vi "LVFunction_Imop_HAS file_GetSoftwareInformation.vi"(0 "HAS file path":path, 11 "error in (no error)":errorcluster) -> (4 "HasoModel":string, 6 "HasoSerial Number":string, 8 "SoftwareOptionsList":string[](array[string]), 13 "comments":string, 14 "session_name":string, 15 "error out":errorcluster)   [LabVIEW 2018]
doc: "Get informations from HasoData object.\n\n<B>HasoDataIn</B> : HasoData object.\n<B>HasoDataOut</B> : HasoData object.\n<B>haso_model</B> : Sensor model.\n<B>haso_serial_number</B> : Haso serial number.\n<B>camera_serial_number</B> : Camera serial number.\n<B>revisions</B> : Revision number.\n<B>lower_calibration_wl</B> : Lower calibration wavelength (nm).\n<B>upper_calibration_wl</B> : Upper calibration wavelength (nm).\n<B>exposure_time_requested</B> : Exposure duration requested, in microsecond.\n<B>exposure_time_applied</B> : Exposure duration applied, in microsecond.\n<B>nb_summed_images</B> : Number of summed images.\n<B>time_stamp</B> : Timestamp.\n<B>is_background_removed</B> : Background removed value.\n<B>is_smearing_removed</B> : Smearing removed value.\n<B>wavelength_nm</B> : Source wavelength (nm).\n<B>session_name</B> : Session name.\n<B>trigger_type</B> : Trigger mode.\n<B>comments</B> : Comments.\n<B>max_level</B> : Max level value.\n<B>start_subpupil</B> : Start subpupil position (um)\n<B>denoising_strength</B> : Sensitivity of spot detection (between 0 and 1). Modulates noise management\n when computing slopes on summed images.\n * 0 : Release constraint on noise to detect as much sub-pupils as possible.\n * 1 : Do not take into account the noise reduction caused by summing.\n<B>ErrorIn </B> : Error\n<B>ErrorOut </B> : Error"
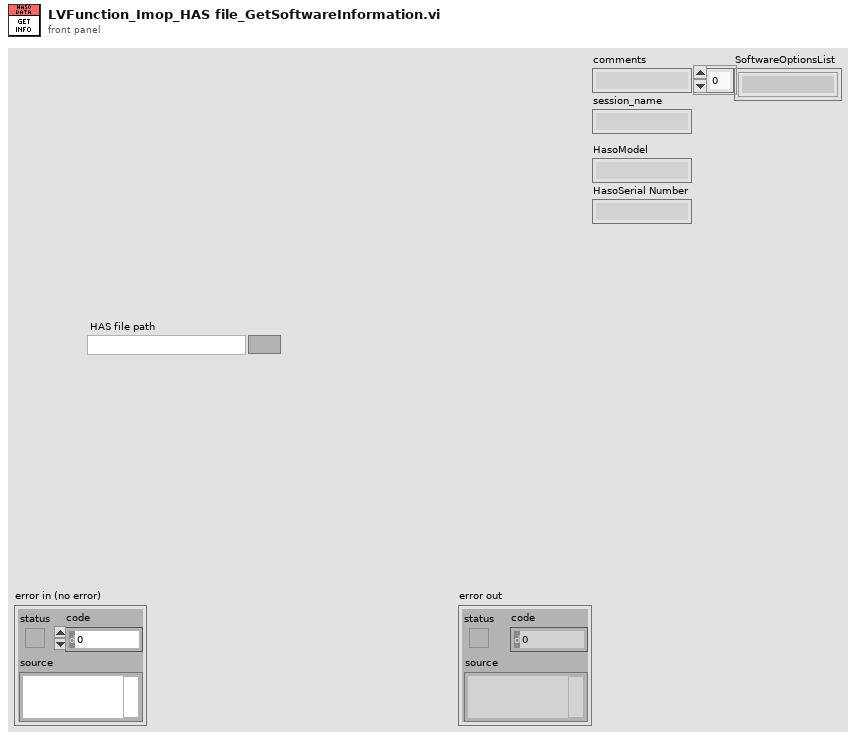
[diagram p1: front panel]
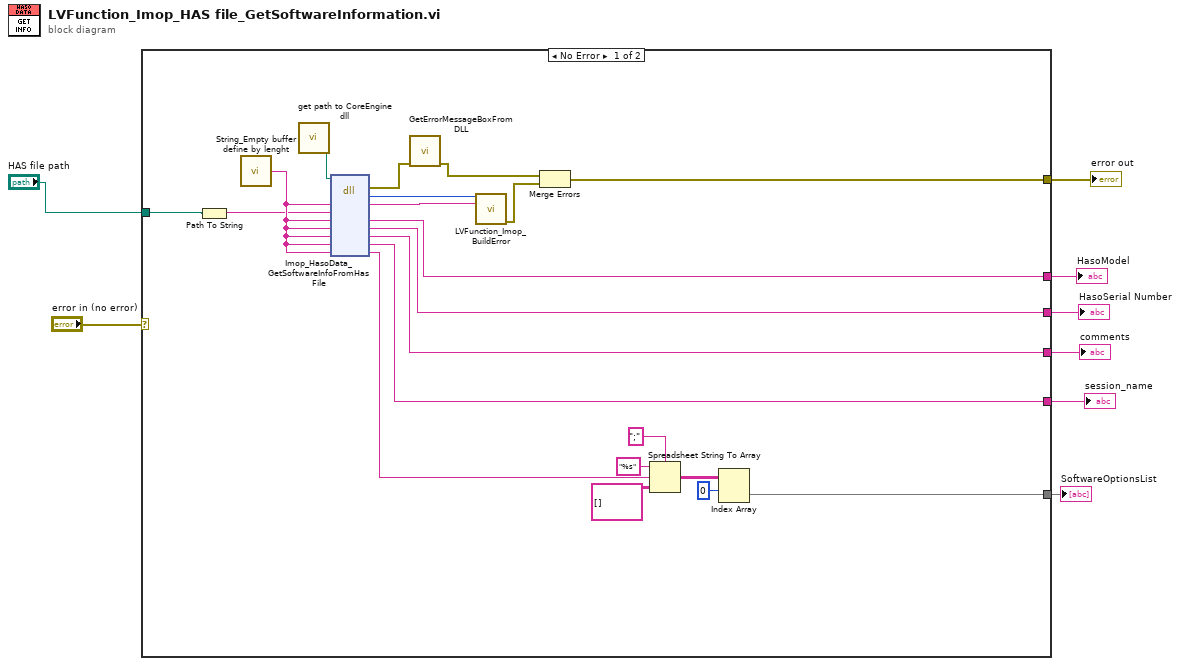
[diagram p0: block diagram]
diagram:
  n1 = case shown="No Error" "error in (no error)" {
    selector: "error in (no error)" -> [_ w30]
    tunnel: [w23 w30] -> w7
    tunnel: [w21 _] -> w6
    tunnel: [w20 _] -> w5
    tunnel: "HAS file path" -> [w19 _]
    tunnel: [w17 _] -> w3
    tunnel: [w16 _] -> w2
    tunnel: [w9 _] -> w1
    frame No Error {
      n2 = Path To String(path=w19) -> (string=w18:string)
      n3 = call "String_Empty buffer define by lenght.vi"() -> ("Empty buffer"=w22:string)  [unwired: 1 in]
      n4 = call "get path to CoreEngine dll.vi"() -> ("path to wavekit library"=w27:path)  [unwired: 14 in, 1 out]
      n5 = dll-call lib="D:/soft/HASO_v3/SVN_trunk/ImOpCoreEngine4_LV2011/DLLs/c_interface_vc100.dll" fn="Imop_HasoData_GetSoftwareInfoFromHasFile"(path in=w27, "message"=w22, "FileName"=w18, "HasoModel"=w22, "HasoSerial Number"=w22, "comments"=w22, "session_name"=w22, "SoftwareInfoList"=w22) -> (error out=w26:errorcluster, "return type"=w29:i32, "message"=w28:string, "HasoModel"=w21:string, "HasoSerial Number"=w20:string, "comments"=w17:string, "session_name"=w16:string, "SoftwareInfoList"=w10:string)  [unwired: 3 in, 1 out]
      n6 = call "GetErrorMessageBoxFromDLL.vi"("error IN"=w26) -> ("error OUT"=w25:errorcluster)  [unwired: 10 in]
      n7 = call "LVFunction_Imop_BuildError.vi"("code"=w29, "String to Prepend to source (\"\")"=w28) -> ("error out"=w24:errorcluster)  [unwired: 13 in]
      n8 = Merge Errors(w25, w24) -> (w23:errorcluster)
      n9 = Spreadsheet String To Array(delimiter (Tab)=";", format string="%s", spreadsheet string=w10, array type (2D Dbl)=string[][] []) -> (array=w14:string[][])
      n10 = Index Array(array=w14, index (row)=0) -> (element=w9:string[])  [unwired: 1 in]
    }
    frame Error {
    }
  }
  "error out" <- w7
  "HasoModel" <- w6
  "HasoSerial Number" <- w5
  "comments" <- w3
  "session_name" <- w2
  "SoftwareOptionsList" <- w1
